vi "Simple Reader.vi"(8 "error in (no error)":errorcluster, 11 "Cryo-Con Driver in":refnum<class "Cryo-Con Driver.lvclass">) -> (0 "error out":errorcluster, 2 "Signals":dbl[](array[numeric]), 3 "Cryo-Con Driver out":refnum<class "Cryo-Con Driver.lvclass">)   [LabVIEW 2016, in "Cryo-Con Driver.lvclass"]
uses:
  Cryo-Con Driver.lvclass
  C:/github/NHMFL_Core/Libraries/Instruments/VISA Instrument/VISA Instrument.lvclass
  C:/github/NHMFL_Core/Libraries/Instruments/Temperature Controller Driver/Temperature Controller Driver.lvclass
  VISA Instrument/VISA Instrument.lvclass/VISA Instrument.ctl
  Temperature Controller Driver/Temperature Controller Driver.lvclass/Temperature Controller Driver.ctl
  VISA Instrument/Read VISA resource.vi
  Temperature Controller Driver/Read T controller configuration.vi
  VISA Instrument/Write VISA resource.vi
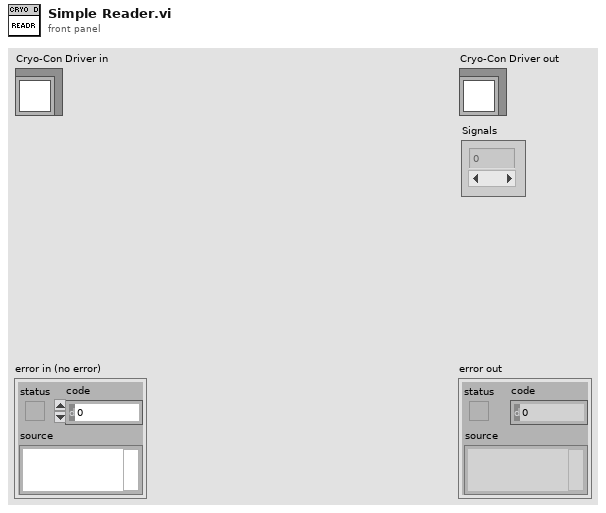
[diagram p1: front panel]
types:
  T1 = typedef "T controller configuration.ctl" = cluster{"Record Channels":string[], "Add raw signal":bool}
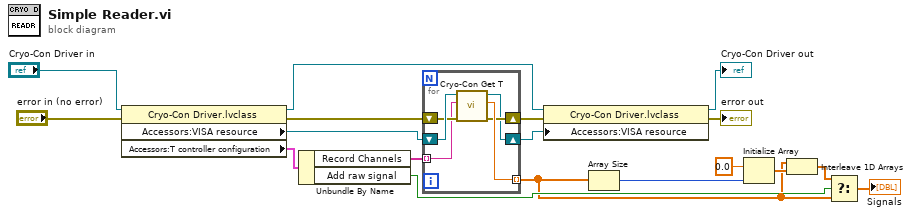
[diagram p0: block diagram]
diagram:
  n1 = property class="Cryo-Con Driver.lvclass"(reference="Cryo-Con Driver in", error in="error in (no error)") -> (reference out=w12:refnum<class "Cryo-Con Driver.lvclass">, error out=w14:errorcluster, "Accessors:VISA resource"=w15:refnum<visa-resource-name>, "Accessors:T controller configuration"=w16:T1)
  n2 = Unbundle By Name(w16) -> ("Record Channels"=w17:string[], "Add raw signal"=w5:bool)
  n3 = for {
    tunnel: w17 -> [w19] mode=indexing
    tunnel: [w22] -> w1 mode=indexing
    shift-right: [w21] -> w8
    shift-left: w14 -> [w23]
    shift-right: [w20] -> w11
    shift-left: w15 -> [w24]
    n4 = call "Cryo-Con Get T.vi"("error in (no error)"=w23, "Channel"=w19, "VISA Resource Name"=w24) -> ("error out"=w21:errorcluster, "Temperature"=w22:dbl, "VISA Resource Name Out"=w20:refnum<visa-resource-name>)  [unwired: 5 in, 1 out]
  }
  n5 = property class="Cryo-Con Driver.lvclass"(reference=w12, error in=w8, "Accessors:VISA resource"=w11) -> (reference out=→"Cryo-Con Driver out":refnum<class "Cryo-Con Driver.lvclass">, error out=→"error out":errorcluster)
  n6 = Array Size(array=w1) -> (size(s)=w7:i32)
  n7 = Initialize Array(0.0 ("element"), w7) -> (w4:dbl[])
  n8 = Interleave 1D Arrays(w1, w4) -> (w3:dbl[])
  n9 = Select(t=w3, s=w5, f=w1) -> (s? t:f=→"Signals":dbl[])
